vi "Laboratory_practice6.vi"() -> ()   [LabVIEW 2022 SP3]
panel:
  out "Peak to Peak":dbl
  in  "stop":bool
  out "RMS":dbl
  out "Waveform Graph":dynamicdata(graph)
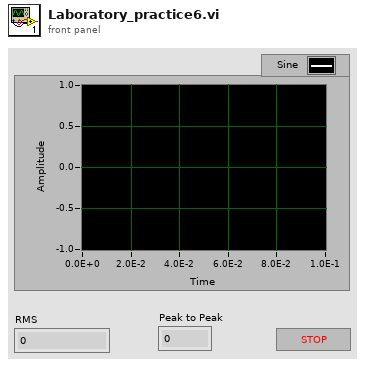
[diagram p1: front panel]
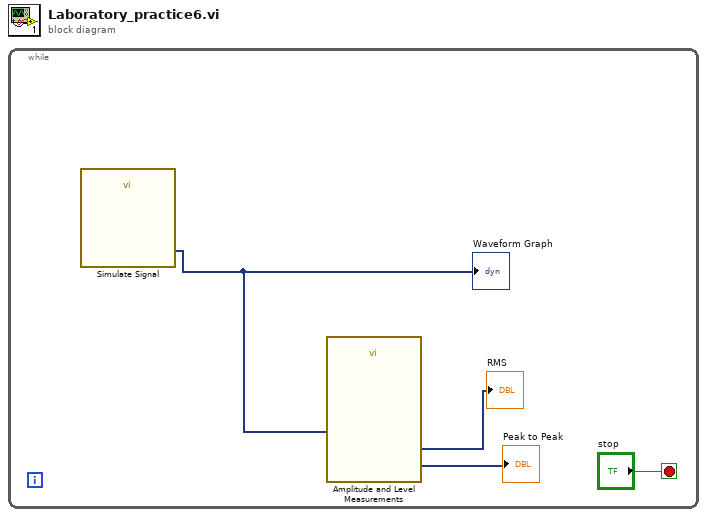
[diagram p0: block diagram]
diagram:
  n1 = while {
    stop <- "stop" stop-if-true
    n2 = call "Simulate Signal"() -> ("Sine"=w2:dynamicdata)  [unwired: 14 in, 1 out]
    "Waveform Graph" <- w2
    n3 = call "Amplitude and Level Measurements"("Signals"=w2) -> ("RMS"=→"RMS":dynamicdata, "Peak to Peak"=→"Peak to Peak":dynamicdata)  [unwired: 12 in, 1 out]
  }
